vi "GUI_Slink_AMP2_3.vi"() -> ()   [LabVIEW 2013]
uses:
  Shared/GUI_Template/GUI_master/tcp_new_data_event.ctl
  Shared/GUI_Template/GUI_master/tcp new data cluster.ctl
  Device Drivers/Gentec Slink/sclae_typdef.ctl
  Shared/Device Driver/OnOffTypeDef.ctl
panel:
  in  "trigger.Channel 2::1":T1 caption="trigger Channel 2"
  in  "trigger.Channel 1::1":T1 caption="Trigger Channel 1"
  in  "Scale.Channel 2::1":T2 caption="Scale PreAmp"
  in  "Scale.Channel 1::1":T2 caption="Scale PreAmp"
  in  "Reading.Channel 2::1":dbl=0.001 caption="AMP3 (J)" min=0.0 max=0.0 format="%_4p"
  in  "stop":bool
  in  "Reading.Channel 1::1":dbl=0.001 caption="AMP2 (J)" min=0.0 max=0.0 format="%_4p"
  in  "GUIdevice 1":string="LB_EnergyMeter_2"
  out "tcp data event":T3
  out "error IO 2":errorcluster
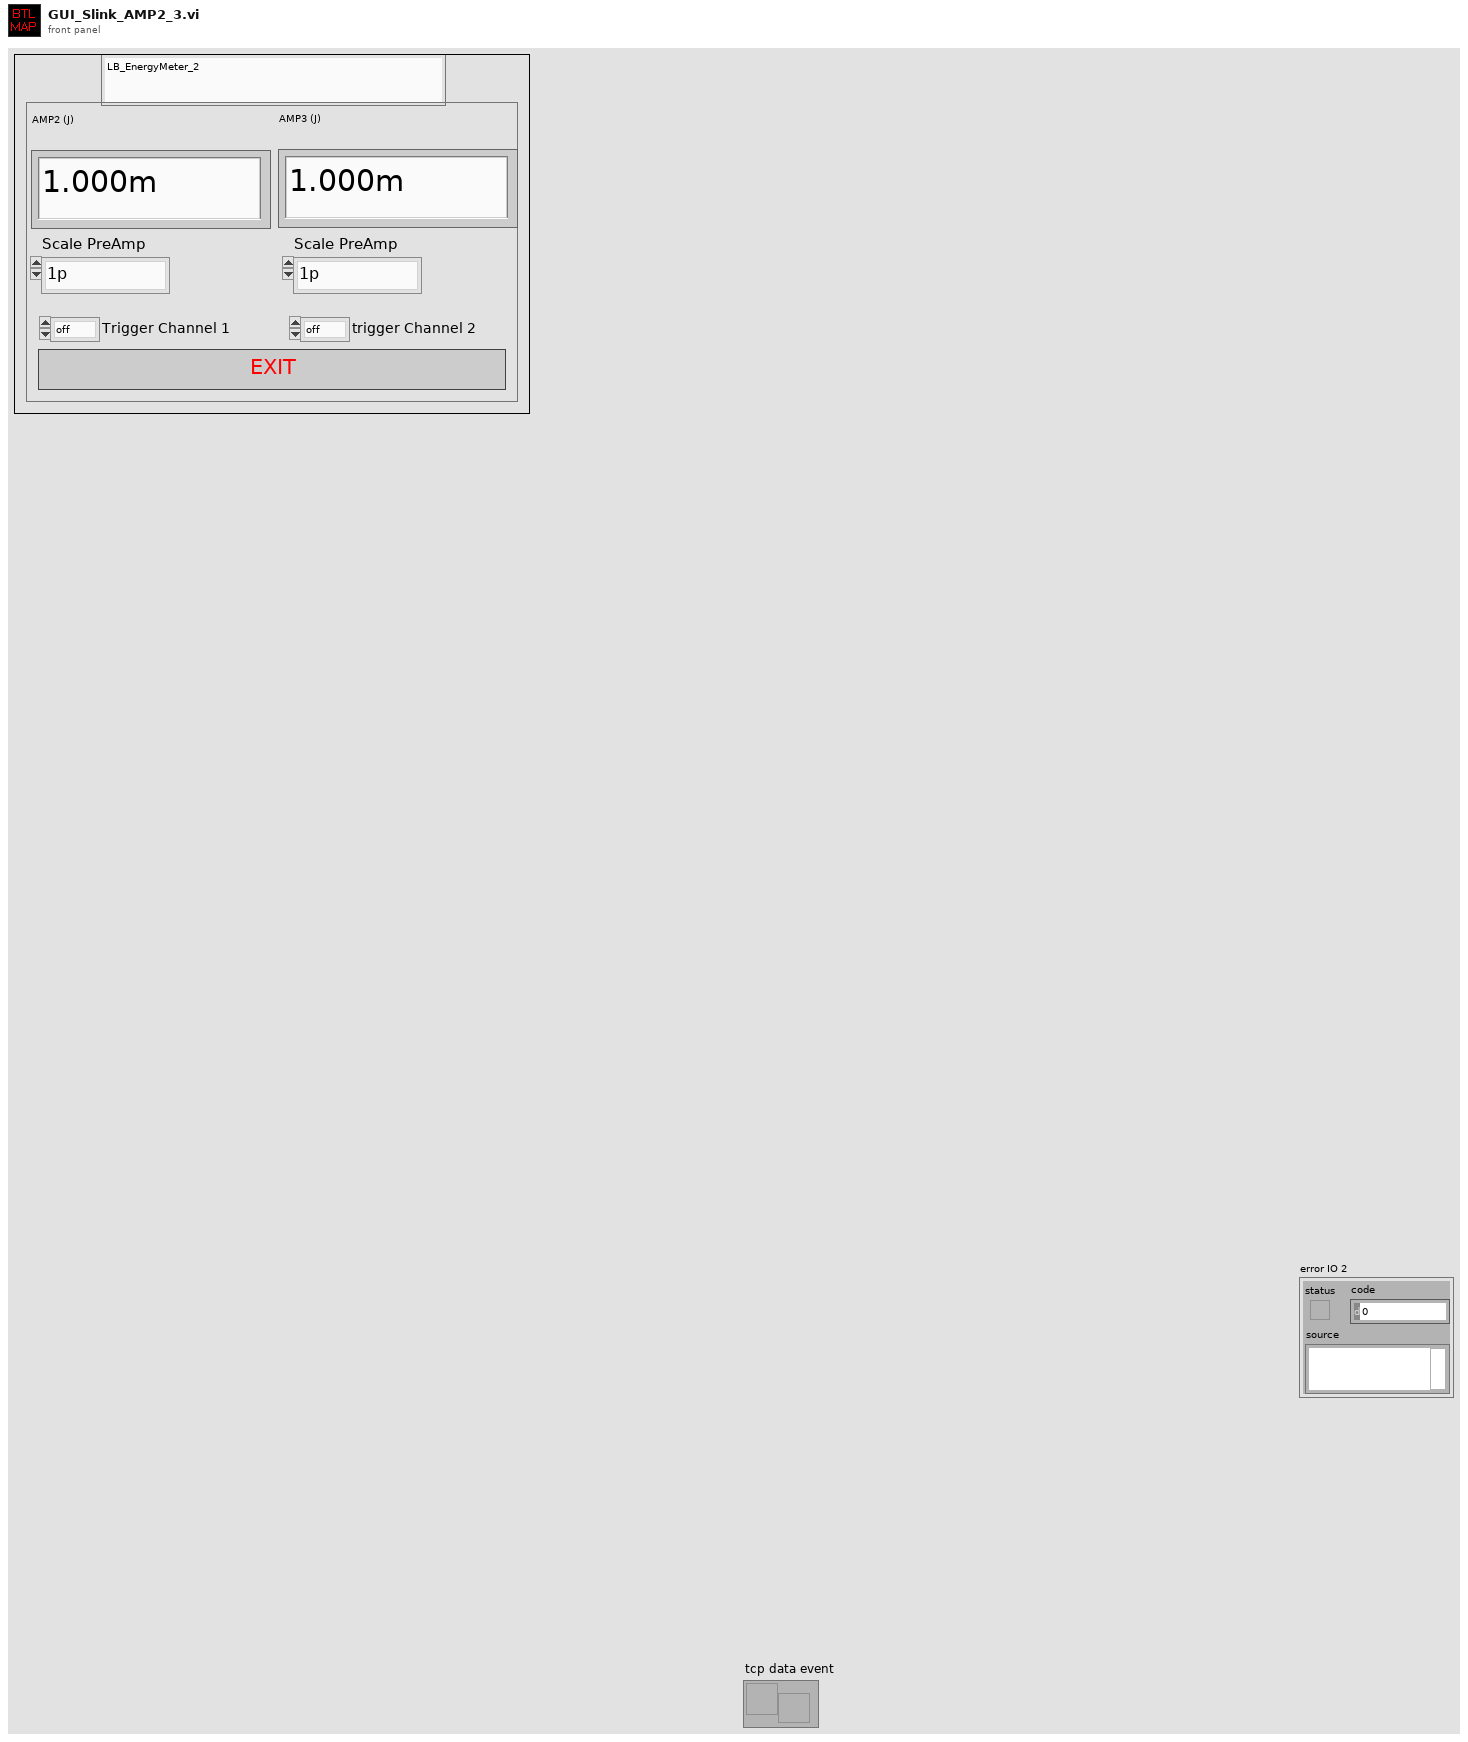
[diagram p1: front panel]
types:
  T1 = typedef "OnOffTypeDef.ctl" = enum16{"off", "on"}
  T2 = typedef "sclae_typdef.ctl" = enum16{"1p", "3p", "10p", "30p", "100p", "300p", "1n", "3n", "10n", "30n", "100n", "300n", "1u", "3u", "10u", "30u", "100u", "300u", "1m", "3m", "10m", "30m", "100m", "300m", "1", "3", "10", "30", "100", "300", "1k", "3k", "10k", "30k", "100k", "300k", "1meg", "3meg", "10meg", "30meg", "100meg", "300meg"}
  T3 = typedef "tcp_new_data_event.ctl" = refnum<user-event>
  T4 = typedef "tcp new data cluster.ctl" = cluster{"EventEnum":enum16{"new data", "connection status update"}, "Device name":string}
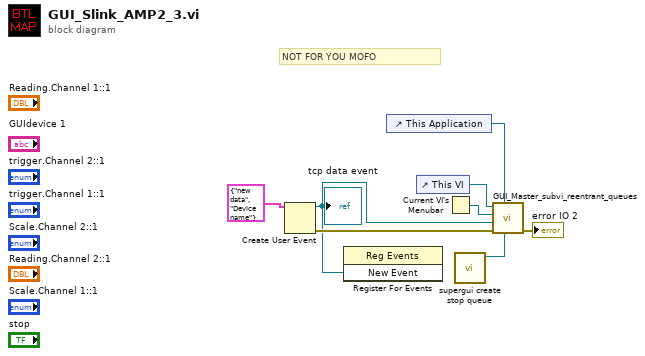
[diagram p0: block diagram]
diagram:
  # "NOT FOR YOU MOFO"
  n1 = Create User Event(user event datatype=T4 {"EventEnum"=enum."new data", "Device name"="Device name"} ("New Event")) -> (user event=w3:refnum<user-event>, error out=w4:errorcluster)  [unwired: 1 in]
  "tcp data event" <- w3
  n2 = register-events(w3) -> ()  [unwired: 2 in, 2 out]
  n3 = control-ref of="This Application"() -> (w2:refnum<vi>)
  n4 = control-ref of="This VI"() -> (w7:refnum<vi>)
  n5 = Current VI's Menubar() -> (w6:refnum<k9>)
  n6 = call "supergui create stop queue.vi"() -> ("STOP Queue out"=w1:refnum<queue>)  [unwired: 11 in]
  n7 = call "GUI_Master_subvi_reentrant_queues.vi"("STOP Queue in"=w1, "This Application"=w2, "error in (no error)"=w4, "tcp data event"=w3, "Caller menu reference"=w6, "Caller VI ref"=w7) -> ("error out"=→"error IO 2":errorcluster)  [unwired: 5 in]
